vi "Transform Vector To Screen Space.vi"() -> ()   [LabVIEW 2022 SP3, in "3D.lvlib"]
uses:
  3D.lvlib
  Vector 3D.ctl
panel:
  in  "a":dbl
  in  "Vector 3D":T1
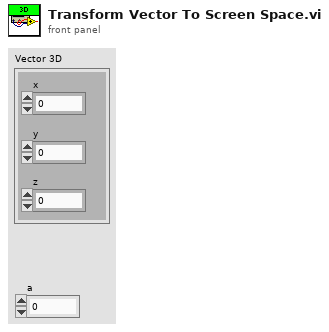
[diagram p1: front panel]
types:
  T1 = typedef "3D.lvlib/Vector 3D.ctl" = cluster{"x":sgl, "y":sgl, "z":sgl}
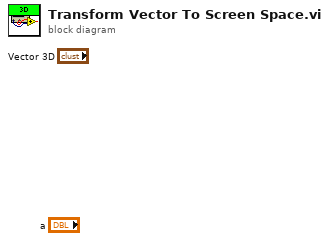
[diagram p0: block diagram]
diagram:
